vi "Abort Download.vi"(8 "error in (no error)":errorcluster, 11 "HTTP GET Async handle":T1) -> (0 "error out":errorcluster, 3 "HTTP GET Async handle out":T1)   [LabVIEW 2019, in "HTTP Client Extensions.lvlib" / "Get Async.lvlib"]
uses:
  Get Async.lvlib
  GET Async.lvclass
  controls/Refnum Type - Enum.ctl
  controls/Refnum Type.ctl
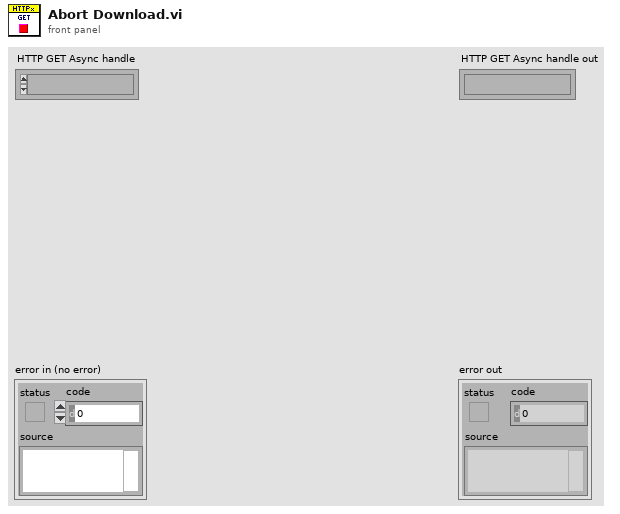
[diagram p1: front panel]
types:
  T1 = typedef "HTTP Client Extensions.lvlib/Get Async.lvlib/Refnum Type.ctl" = refnum<k1>
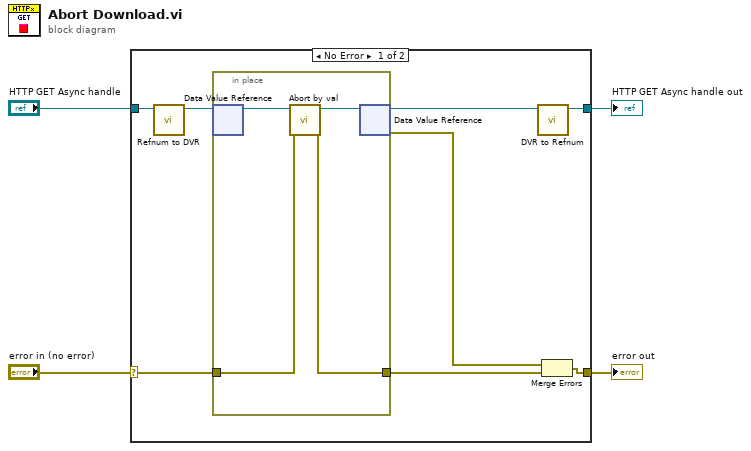
[diagram p0: block diagram]
diagram:
  n1 = case shown="No Error" "error in (no error)" {
    selector: "error in (no error)" -> [w12 w18]
    tunnel: [w10 w18] -> w3
    tunnel: [w7 w17] -> w1
    tunnel: "HTTP GET Async handle" -> [w5 w17]
    frame No Error {
      n2 = call "Refnum to DVR.vi"("Refnum out"=w5) -> ("Data Value Reference in"=w6:refnum<data-value>)  [unwired: 10 in]
      n3 = in-place {
        in-place-border: w12 -> [w13]
        in-place-border: [w14] -> w11
        n4 = in-place-dvr #1(w6) -> (w16:refnum<class "GET Async.lvclass">)  [unwired: 1 out]
        n5 = call "Abort by val.vi"("error in (no error)"=w13, "HTTP GET Async.lvclass"=w16) -> ("error out"=w14:errorcluster, "HTTP GET Async.lvclass out"=w15:refnum<class "GET Async.lvclass">)  [unwired: 8 in]
        n6 = in-place-dvr #1(w15) -> (w8:refnum<data-value>, w9:errorcluster)
      }
      n7 = call "DVR to Refnum.vi"("Data Value Reference in"=w8) -> ("Refnum out"=w7:T1)  [unwired: 10 in]
      n8 = Merge Errors(w9, w11) -> (w10:errorcluster)
    }
    frame Error {
    }
  }
  "error out" <- w3
  "HTTP GET Async handle out" <- w1
